vi "image recorder main panel.vi"() -> ()   [LabVIEW 2021]
uses:
  <vilib>/Utility/error.llb/DialogType.ctl
  Image-Stack-Compressor/StackWriterWrapper/LV code/StackWriterWrapper.lvlib
  <vilib>/ptbypt/NI_PtbyPt.lvlib
panel:
  in  "allow long names":bool
  in  "use short dir":bool=TRUE
  out "characters in file name":i32
  in  "Experimenter Name":string
  in  "load control values from file":bool
  in  "save control values to file":bool
  in  "Edit":bool[](array[boolean])
  in  "Add Stimulus":bool
  in  "Delete":bool[](array[boolean])
  out "stimulii":string[](array[string])
  in  "Training/Habituation Pre Exposure":T1
  in  "Stimulus Array":T2(array[cluster])
  in  "Genotype":T3={"GAL4 Line / Line A / Genotype"="CS", "UAS-Effector Line / Line B"=""}
  in  "Project":string
  out "frame add time":u32
  out "last loop time":u32
  in  "left of screen":string="air inlet"
  in  "bottom of screen":string="CS"
  in  "top of screen":string="back of box (y = 0)"
  in  "central region (frac)":dbl caption="central region for placement\nsize (fraction of full screen)"
  out "loop time":u32
  in  "max Background Compression Threads":i32=4
  in  "maxBytesToWrite":u64=1950000000 format="%.2p"
  in  "limit file size?":bool
  out "notes last updated":timestamp format="%<%I:%M %p\n%d/%m/%y>T"
  in  "notes":string
  out "avg frame rate (fps)":dbl
  out "total loop\nwith delay":u32
  out "delay time":dbl
  in  "auto-set":bool
  out "numToWrite":i32(slide) scale=0.0..10.0
  out "numToCompress":i32(slide)=1 scale=0.0..10.0
  out "loop too fast":bool
  in  "min loop time (ms)":u32
  out "timing report":string="-\n  name: adding frame to stack\n  ncalls: 72\n  totaltime: 0.298202\n  maxtime: 0.00436328\n  mintime: 0.00225001\n  avg time: 0.00414169\n  numblowntics: 0\n-\n  name: cloning image\n  ncalls: 72\n  totaltime: 0.24642\n  maxtime: 0.00378184\n  mintime: 0.0017782\n  avg time: 0.0034225\n  numblowntics: 0\n-\n  name: compressing a frame\n  ncalls: 72\n  totaltime: 1.94123\n  maxtime: 0.0403699\n  mintime: 0.0239481\n  avg time: 0.0269615\n  numblowntics: 0\n-\n  name: creating save description\n  ncalls: 1\n  totaltime: 6.19014e-005\n  maxtime: 6.19014e-005\n  mintime: 6.19014e-005\n  avg time: 6.19014e-005\n  numblowntics: 0\n-\n  name: deleting written stack from memory\n  ncalls: 1\n  totaltime: 0.00222322\n  maxtime: 0.00222322\n  mintime: 0.00222322\n  avg time: 0.00222322\n  numblowntics: 0\n-\n  name: writing a stack to disk\n  ncalls: 1\n  totaltime: 0.0259505\n  maxtime: 0.0259505\n  mintime: 0.0259505\n  avg time: 0.0259505\n  numblowntics: 0\ncxcore: 1.0.0, cv: 1.0.0\n\n"
  out "stack destination":string="C:\\data\\test\\t10\\n#n#n#n\\CS(CS)\\2011\\09\\14\\1334\\CS@CS@t10@n#n#n#n@30.mmf"
  out "stackwriter pointer":u32=314603384
  out "loop iteration":i32=23494
  out "error out":errorcluster
  out "maximum loop time":u32
  out "average loop time":dbl format="%.2p"
  in  "max stack size":dbl=1.99
  out "GB written":dbl format="%.2f"
  out "max file size in GB":u64=8589934591
  out "MB written":i32
  out "average time to compress a frame":dbl format="%#_3p"
  out "average time to add a frame to stack":dbl format="%#_3p"
  out "average time to write a stack":dbl format="%#_3p"
  out "elapsed time(s)":dbl
  in  "anticipated frame rate":dbl=30.0
  in  "lgDimMinSize":i32=5
  in  "keyFrameInterval":i32=90
  in  "smallDimMinSize":i32=3
  in  "thresholdAboveBackground":i32=7
  out "buffer number":u32
  in  "base directory":path=path "C:/data/test"
  out "filename":string="CS@CS@t10@n#n#n#n@30"
  out "data directory":path=path "C:/data/test/t10/n#n#n#n/CS(CS)/2011/09/14/1334"
  in  "setup camera?":bool
  in  "STOP PROGRAM":bool
  in  "STOP ACQUISITION":bool
  in  "MAKE DIRECTORIES":bool
  in  "START ACQUISITION":bool
  in  "use ROI":bool
  in  "region of interest":cluster{"x0":u32, "y0":u32, "w":u32, "h":u32}={"x0"=0, "y0"=0, "w"=5000, "h"=5000}
  in  "Acquisiton Time (s)":dbl=660.0
  in  "update image every __ ms":u16=500
  out "Camera Image":T4(plugin-control)
  in  "set all control values as default":bool
  out "GAL4 Line":string="CS"
  # "to reset to actual defaults, delete file\nimage recorder main panel ctl values.dflt"
  # "MMF compression settings"
  # "debugging stuff"
  # "X"
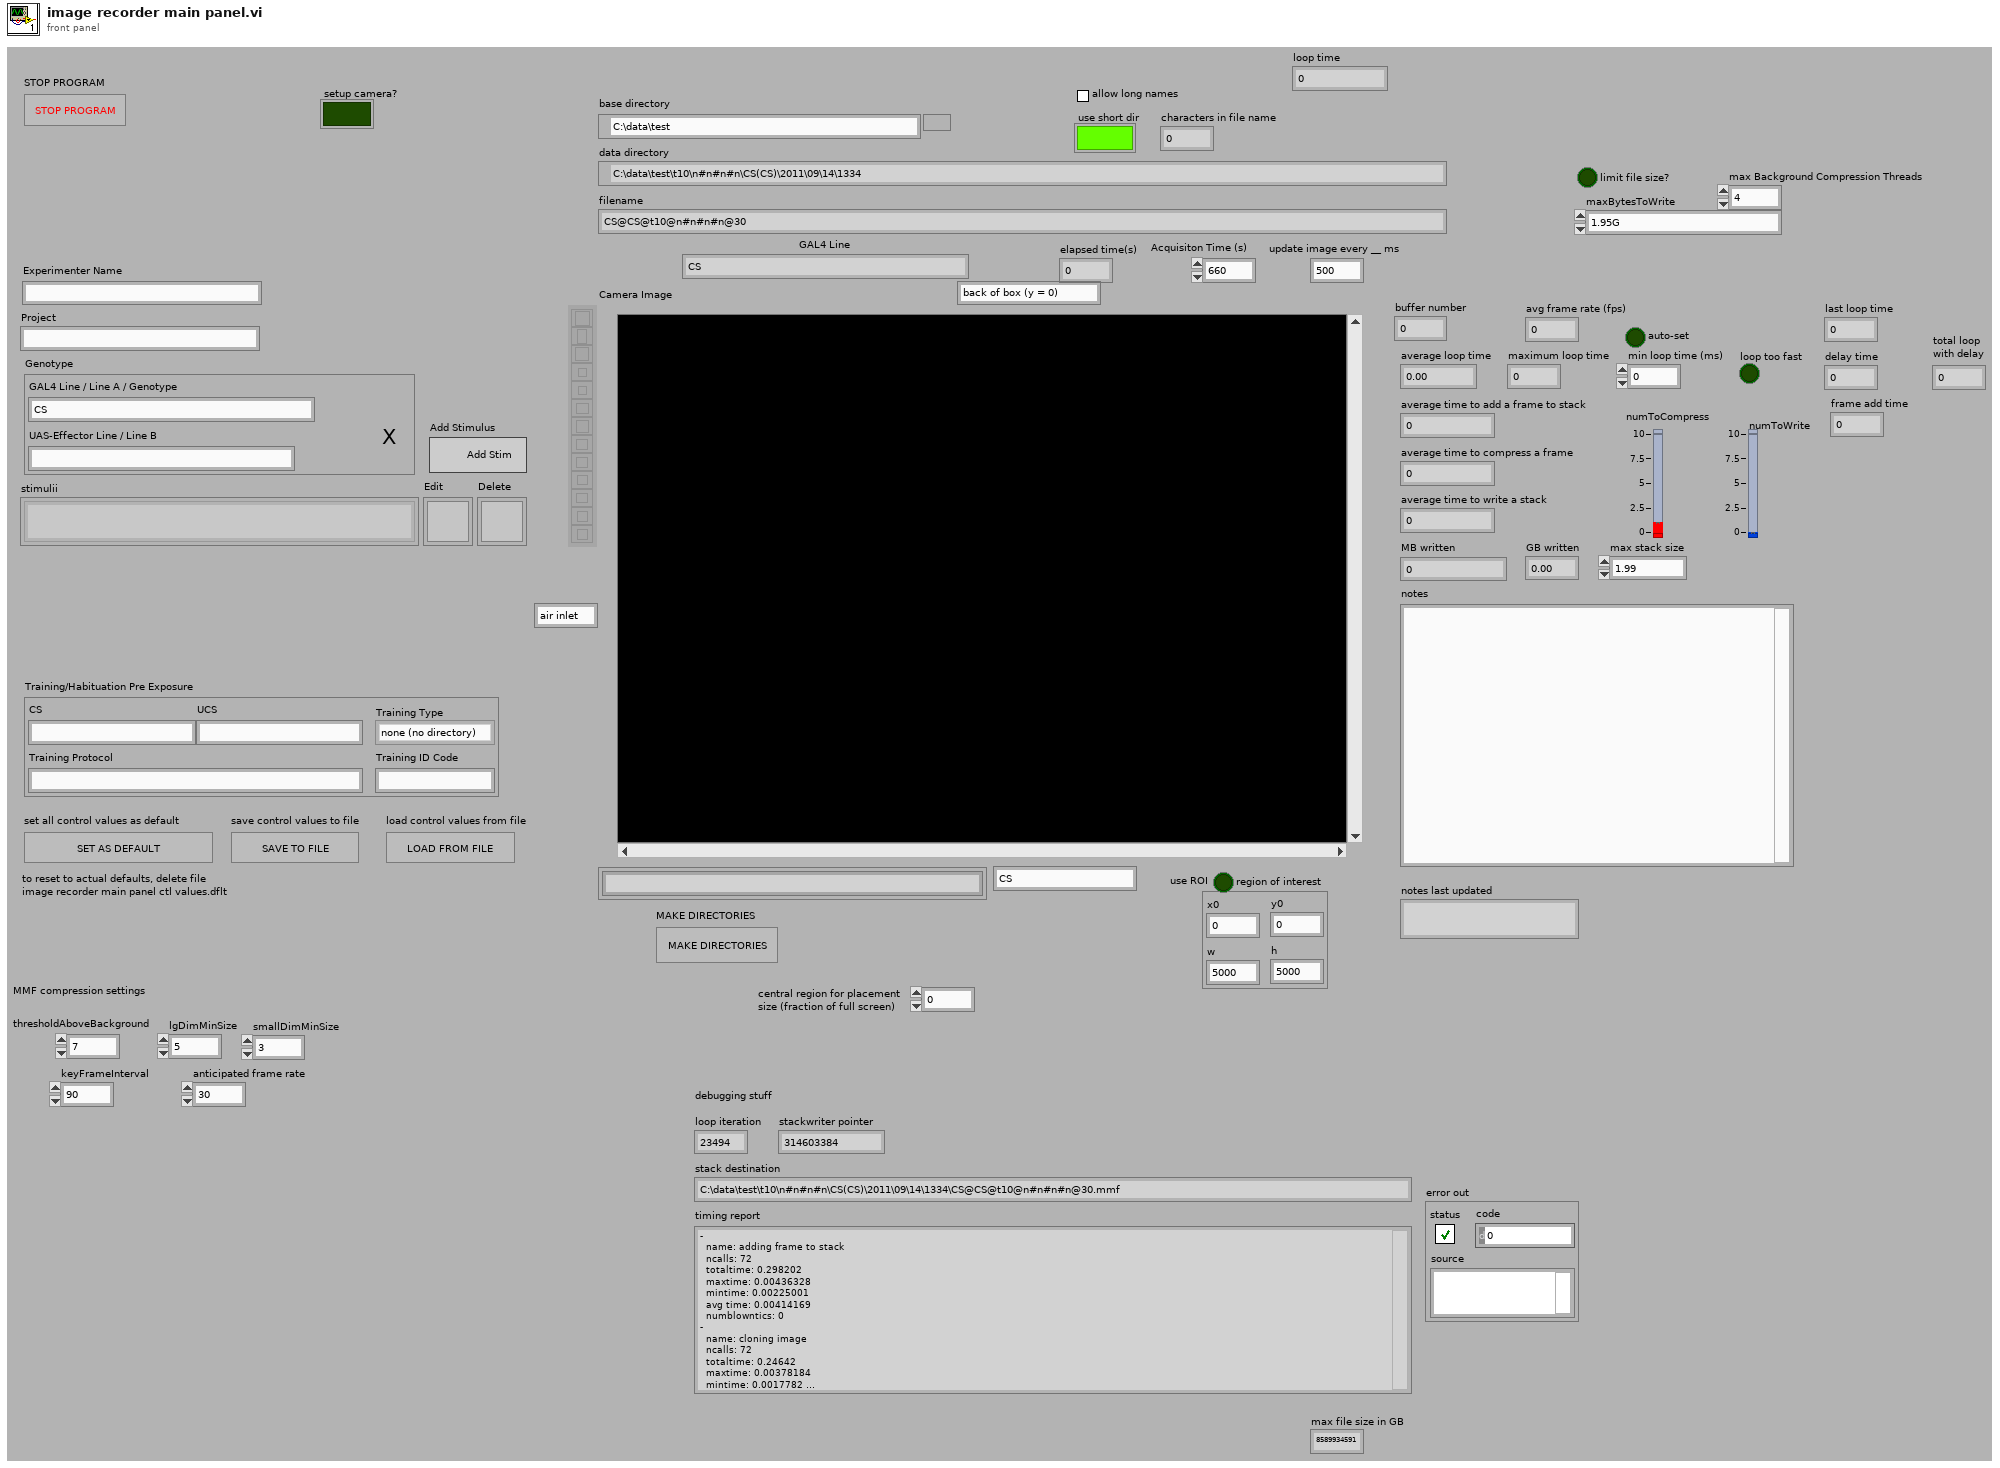
[diagram p1: front panel]
types:
  T1 = cluster{"CS":string, "UCS":string, "Training Protocol":string, "Training ID Code":string, "Training Type":enum16{"none (no directory)", "habituated", "mock habituated", "untrained", "trained"}}
  T2 = cluster{"Stimulus Structure":enum16{"Noise", "Temporal", "Spatial", "Constant", "Other"}, "Stimulant":enum16{"Red Light", "Blue Light", "Green Light", "Odor", "Temperature", "Taste", "Other"}, "Stimulant - additional detail":string, "Noise Parameters":cluster{"Min Val":dbl, "Noise Type":enum16{"Brownian", "Gaussian", "M-Sequence", "Integral of M-Sequence", "Bernoulli", "Uniform", "Other"}, "Max Val":dbl, "Sigma \n(For Gaussian/Brownian)":dbl, "Update Rate (Hz)":dbl, "Full Scale Intensity \n(detector Watts)":dbl, "additional string to append":string, "Other Noise Type":string}, "Temporal Parameters":cluster{"maximum":dbl, "mimimum":dbl, "period (s)":dbl, "Temporal Pattern":enum16{"Triangle", "Sine", "Square", "Other"}, "unit":string, "additional string to append":string, "other pattern":string}, "Spatial Parameters":cluster{"maximum":dbl, "mimimum":dbl, "distance":dbl, "Spatial Pattern":enum16{"XLinear", "YLinear", "Droplet", "Radial", "Other"}, "unit":string, "period_unit":string, "additional string to append":string, "other pattern":string}, "Constant Parameters":cluster{"Value":dbl, "unit":string, "additional string to append":string}, "Other Parameters":cluster{"Long Description of Stimulus And Parameters":string, "Short Description for File Name":string}}[]
  T3 = cluster{"GAL4 Line / Line A / Genotype":string, "UAS-Effector Line / Line B":string}
  T4 = typedef "IMAQ Image.ctl" = refnum<image>
  T5 = typedef "DialogType.ctl" = u16
  T6 = typedef "IMAQdx.ctl" = refnum<k21>
  T7 = cluster{"Aquisition Type":enum16{"IMAQ", "IMAQdx", "AVI", "MMF", "STACK"}, "Interface Name":string, "use roi":bool, "ROI":cluster{"left":u16, "top":u16, "width":u16, "height":u16}, "camera name":T6, "AVI Path":path, "mmf path":path, "stub":string, "Field Width (0 disables 0 padding)":u8, "extension":string, "inter-frame interval (ms)":dbl}
  T8 = typedef "AviRefnum.ctl" = refnum<k1>
  T9 = cluster{"Aquisition Type":enum16{"IMAQ", "IMAQdx", "AVI", "MMF", "STACK"}, "IMAQ Session Out":refnum<k11>, "imaqdx session":T6, "AVI parameters":cluster{"Avi Refnum ":T8, "inter-frame interval (ms)":dbl}, "mmf parameters":cluster{"mmf pointer":u32, "inter-frame interval (ms)":dbl}, "stack read info":cluster{"file stub":string, "format string":string, "extension":string, "inter-frame interval (ms)":dbl}, "camera image":T4, "camera image is 8 bit":bool, "8 bit camera image":T4}
  T10 = enum16{"Reset Table", "Get Values", "Add Value", "Get Table", "Get Spreadsheet", "set stack writer"}
  T11 = enum16{"open", "replace", "create", "open or create", "replace or create", "replace or create with confirmation"}
  T12 = cluster{"Stimulus Structure":enum16{"Noise", "Temporal", "Spatial", "Constant", "Other"}, "Stimulant":enum16{"Red Light", "Blue Light", "Green Light", "Odor", "Temperature", "Taste", "Other"}, "Stimulant - additional detail":string, "Noise Parameters":cluster{"Min Val":dbl, "Noise Type":enum16{"Brownian", "Gaussian", "M-Sequence", "Integral of M-Sequence", "Bernoulli", "Uniform", "Other"}, "Max Val":dbl, "Sigma \n(For Gaussian/Brownian)":dbl, "Update Rate (Hz)":dbl, "Full Scale Intensity \n(detector Watts)":dbl, "additional string to append":string, "Other Noise Type":string}, "Temporal Parameters":cluster{"maximum":dbl, "mimimum":dbl, "period (s)":dbl, "Temporal Pattern":enum16{"Triangle", "Sine", "Square", "Other"}, "unit":string, "additional string to append":string, "other pattern":string}, "Spatial Parameters":cluster{"maximum":dbl, "mimimum":dbl, "distance":dbl, "Spatial Pattern":enum16{"XLinear", "YLinear", "Droplet", "Radial", "Other"}, "unit":string, "period_unit":string, "additional string to append":string, "other pattern":string}, "Constant Parameters":cluster{"Value":dbl, "unit":string, "additional string to append":string}, "Other Parameters":cluster{"Long Description of Stimulus And Parameters":string, "Short Description for File Name":string}}
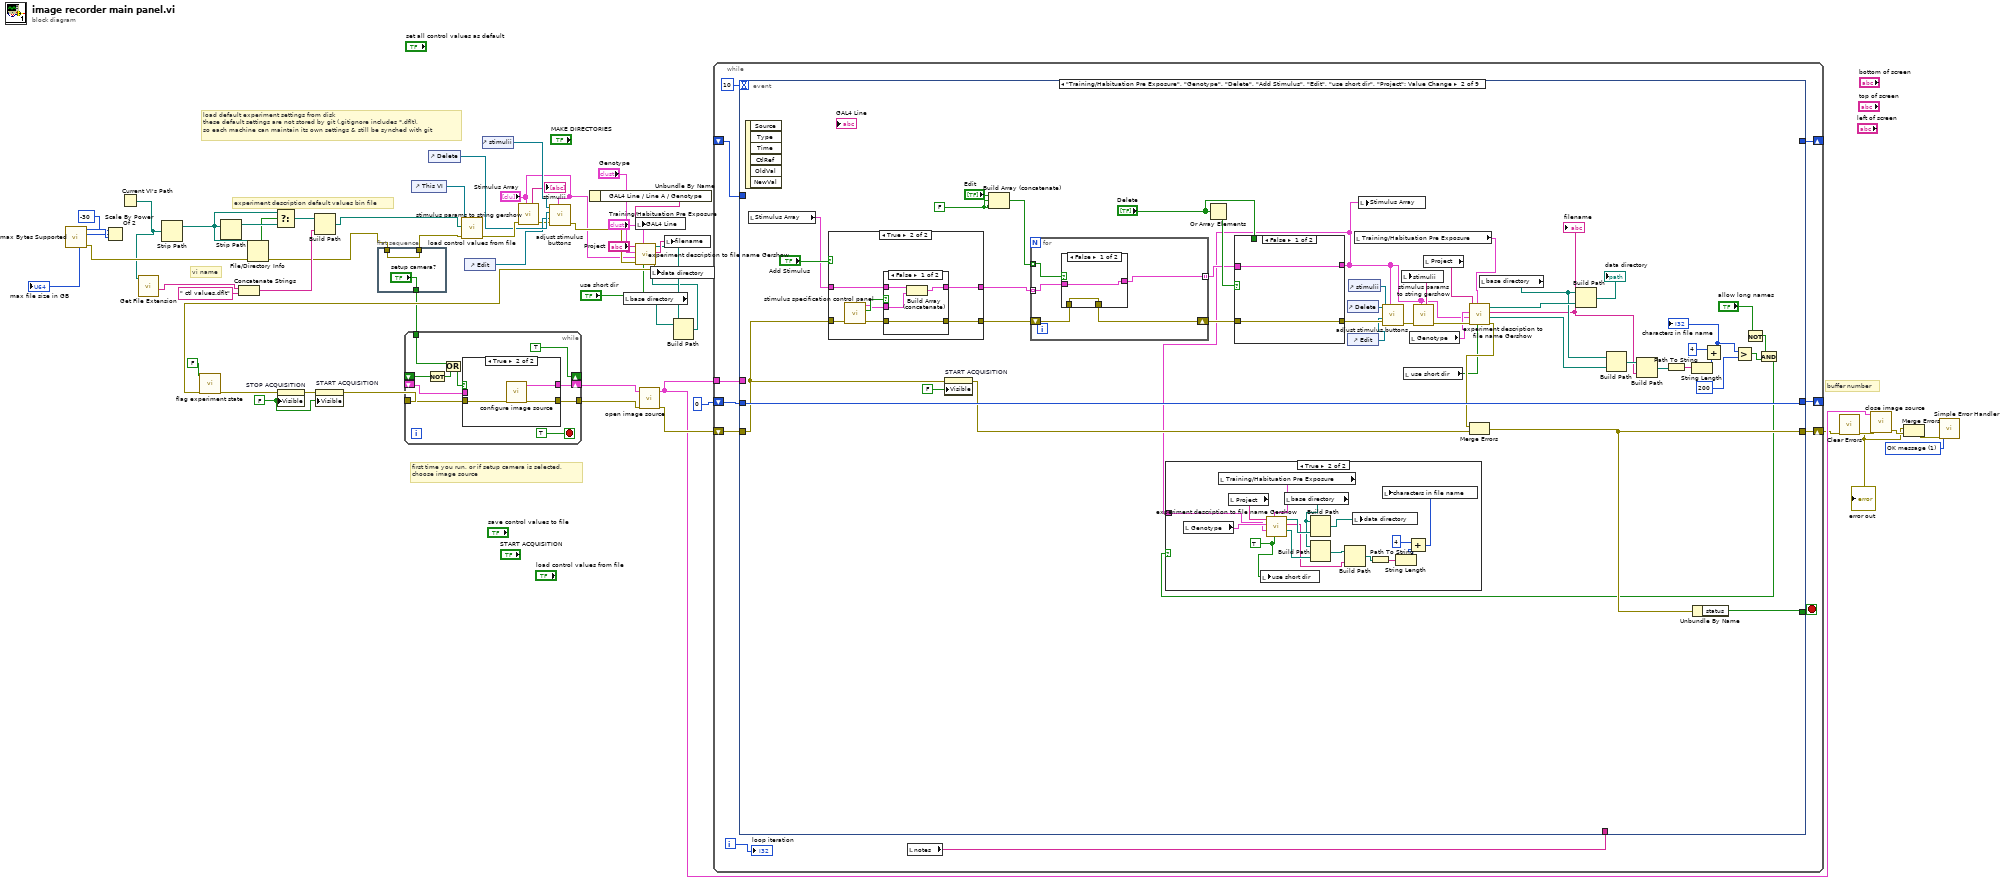
[diagram p0: block diagram]
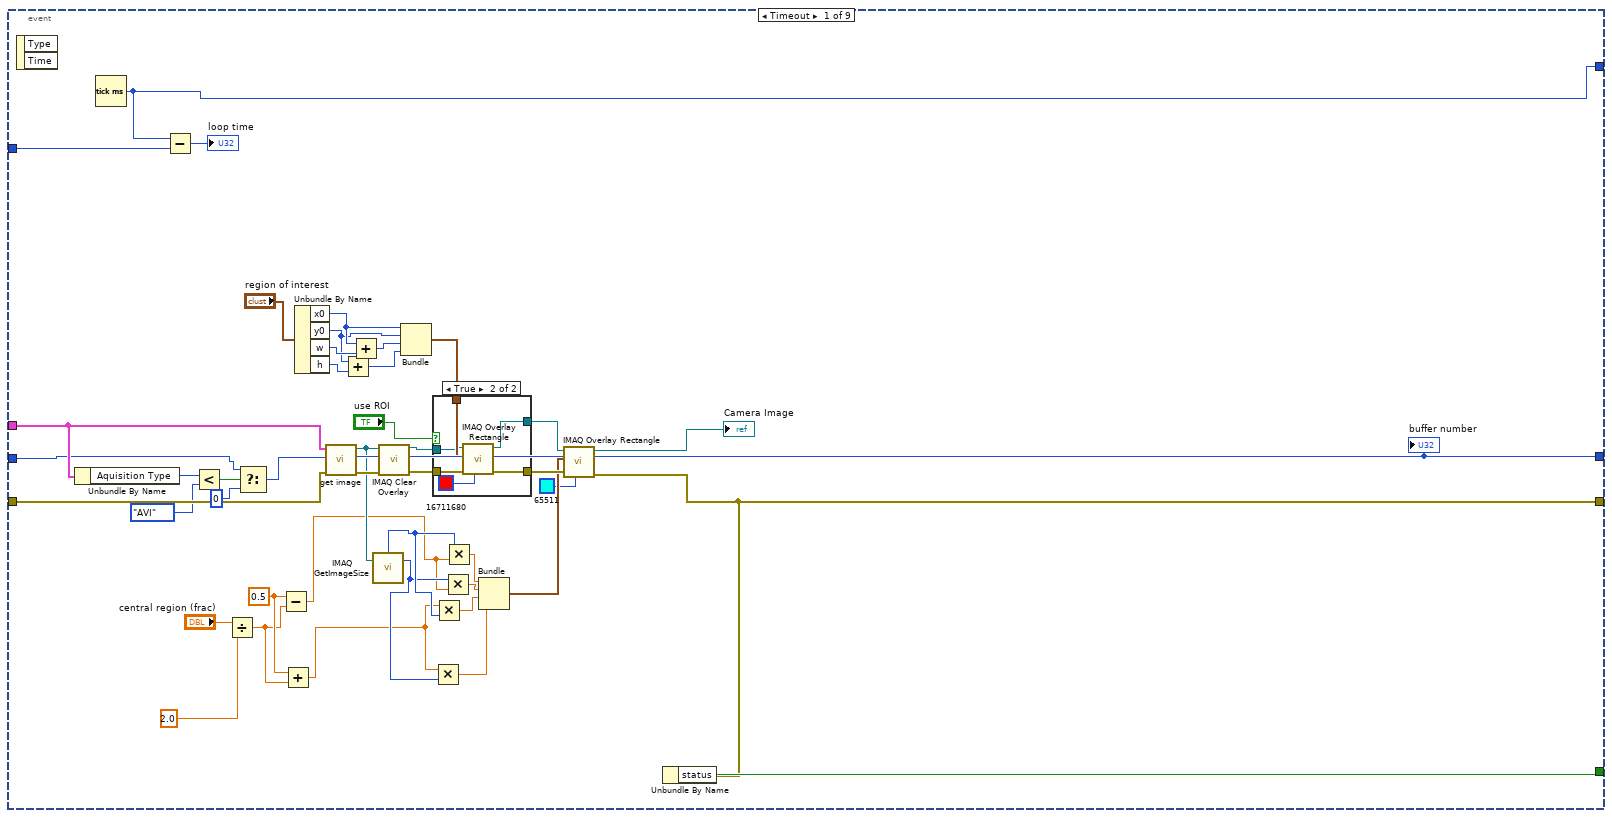
[diagram p3: hidden frame]
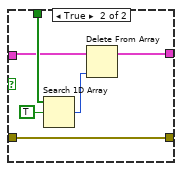
[diagram p6: hidden frame]
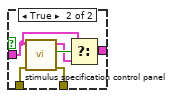
[diagram p7: hidden frame]
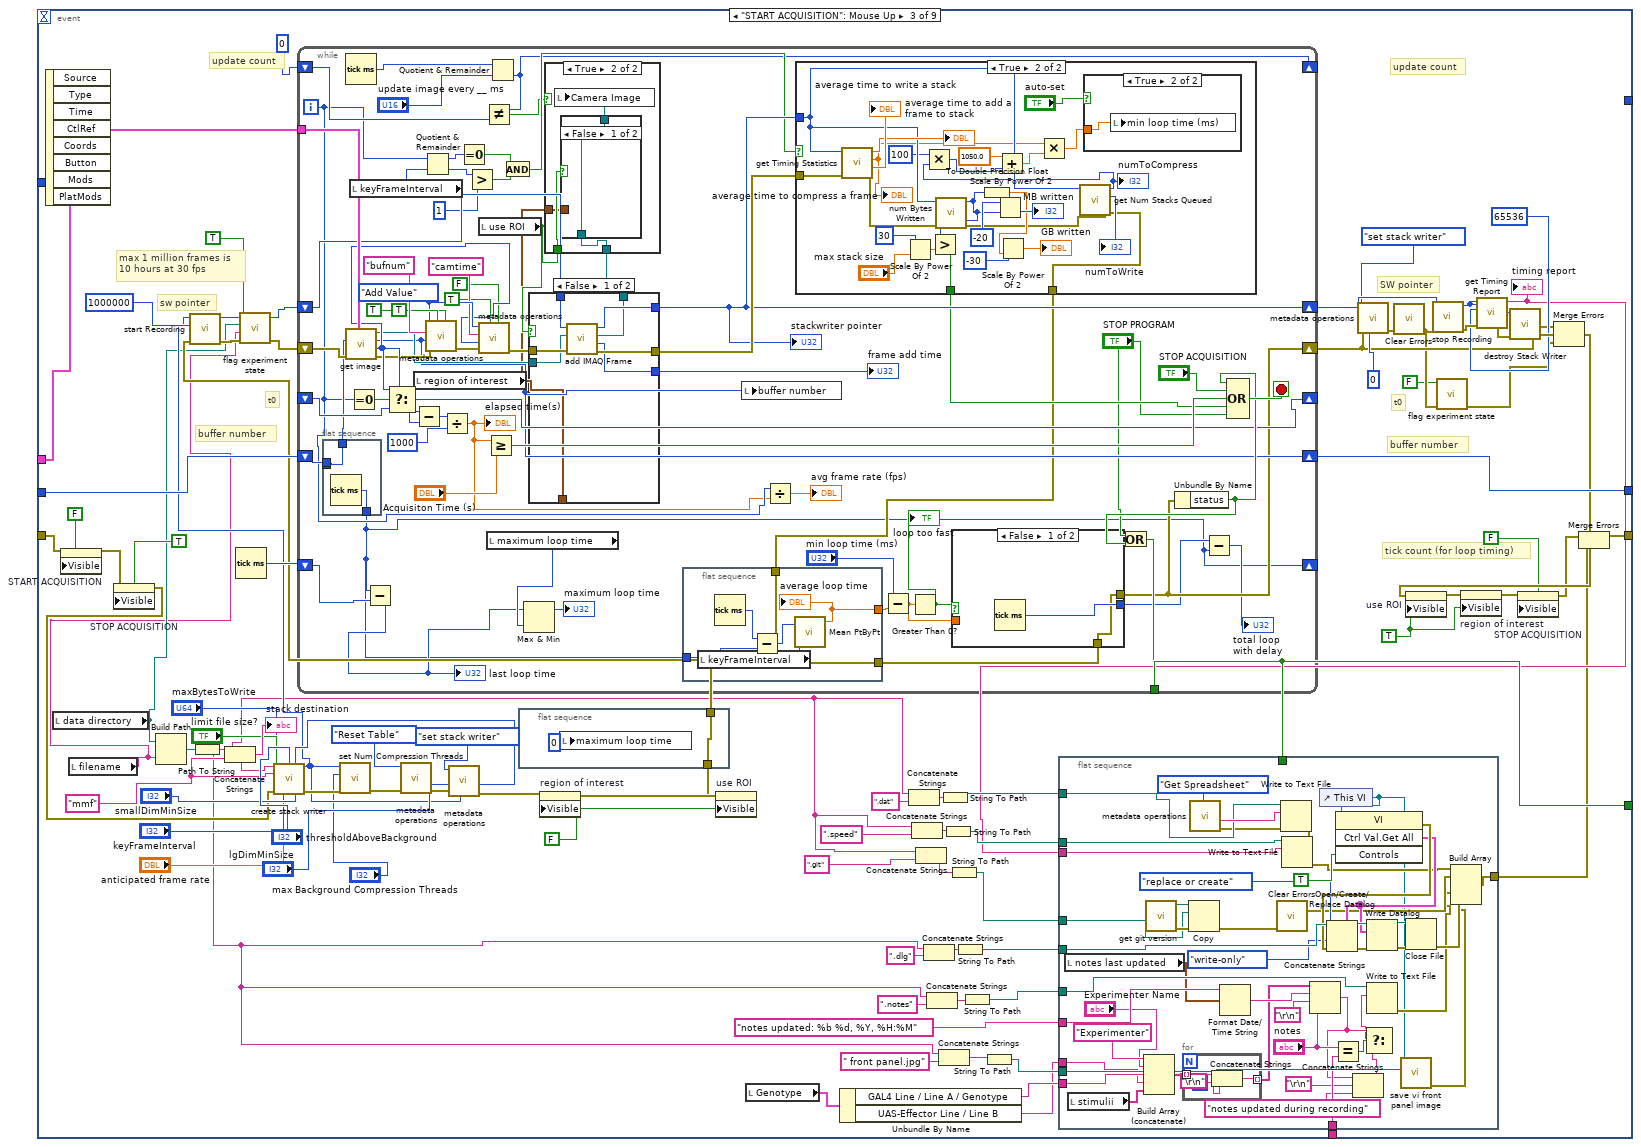
[diagram p10: hidden frame]
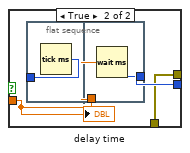
[diagram p11: hidden frame]
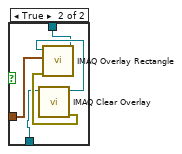
[diagram p13: hidden frame]
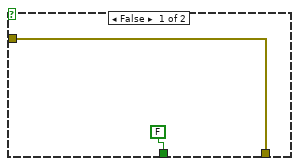
[diagram p14: hidden frame]
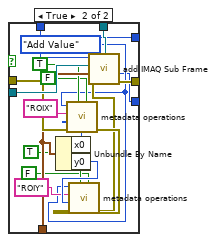
[diagram p16: hidden frame]
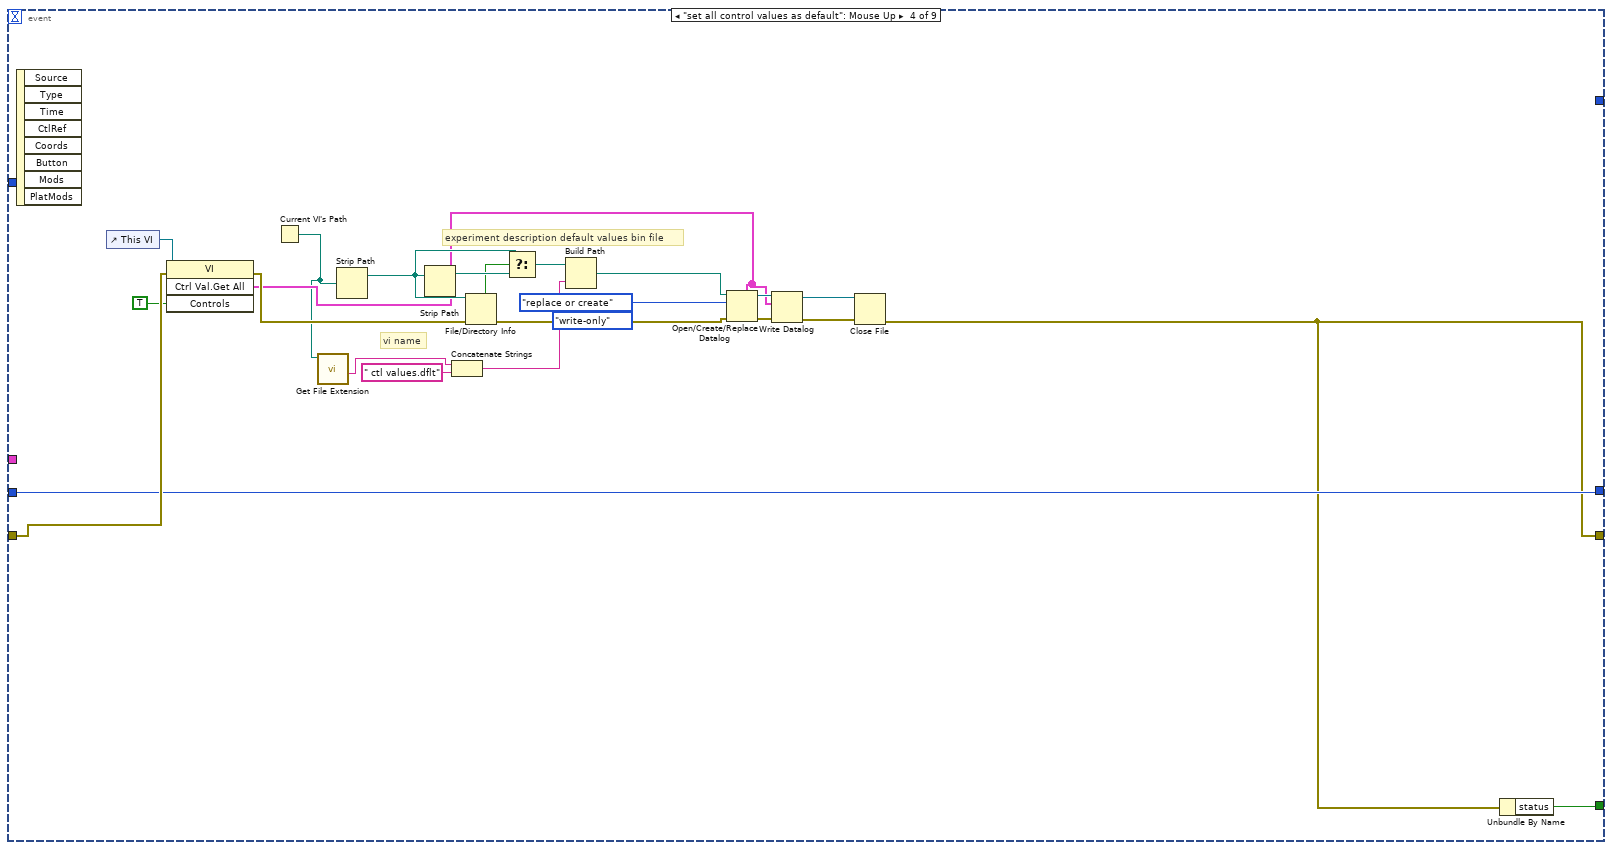
[diagram p17: hidden frame]
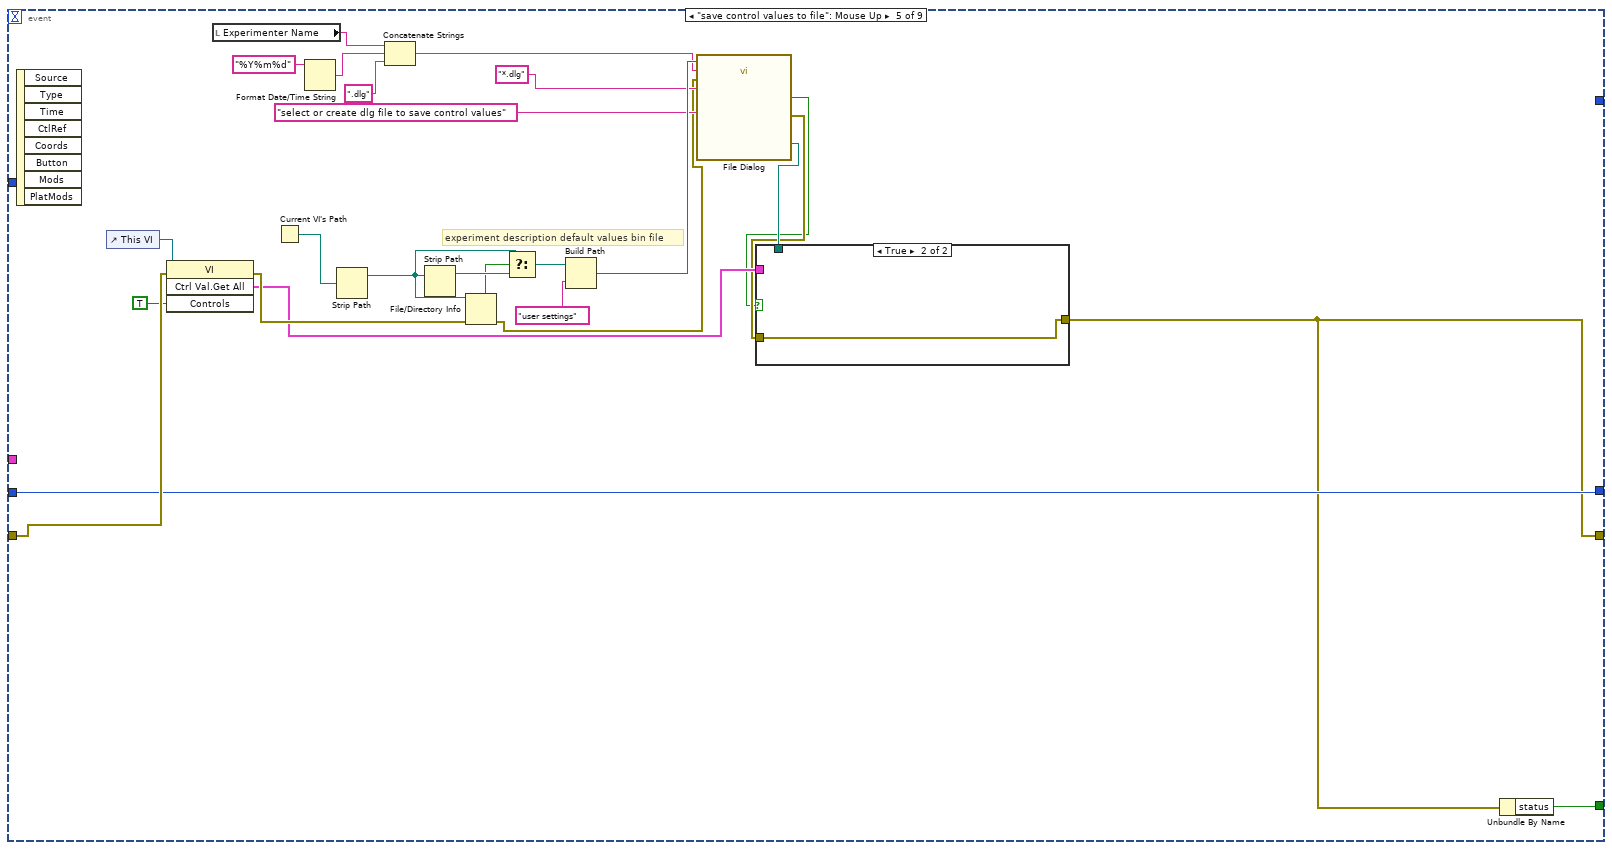
[diagram p18: hidden frame]
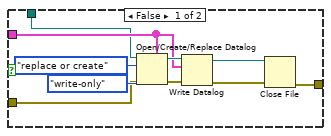
[diagram p19: hidden frame]
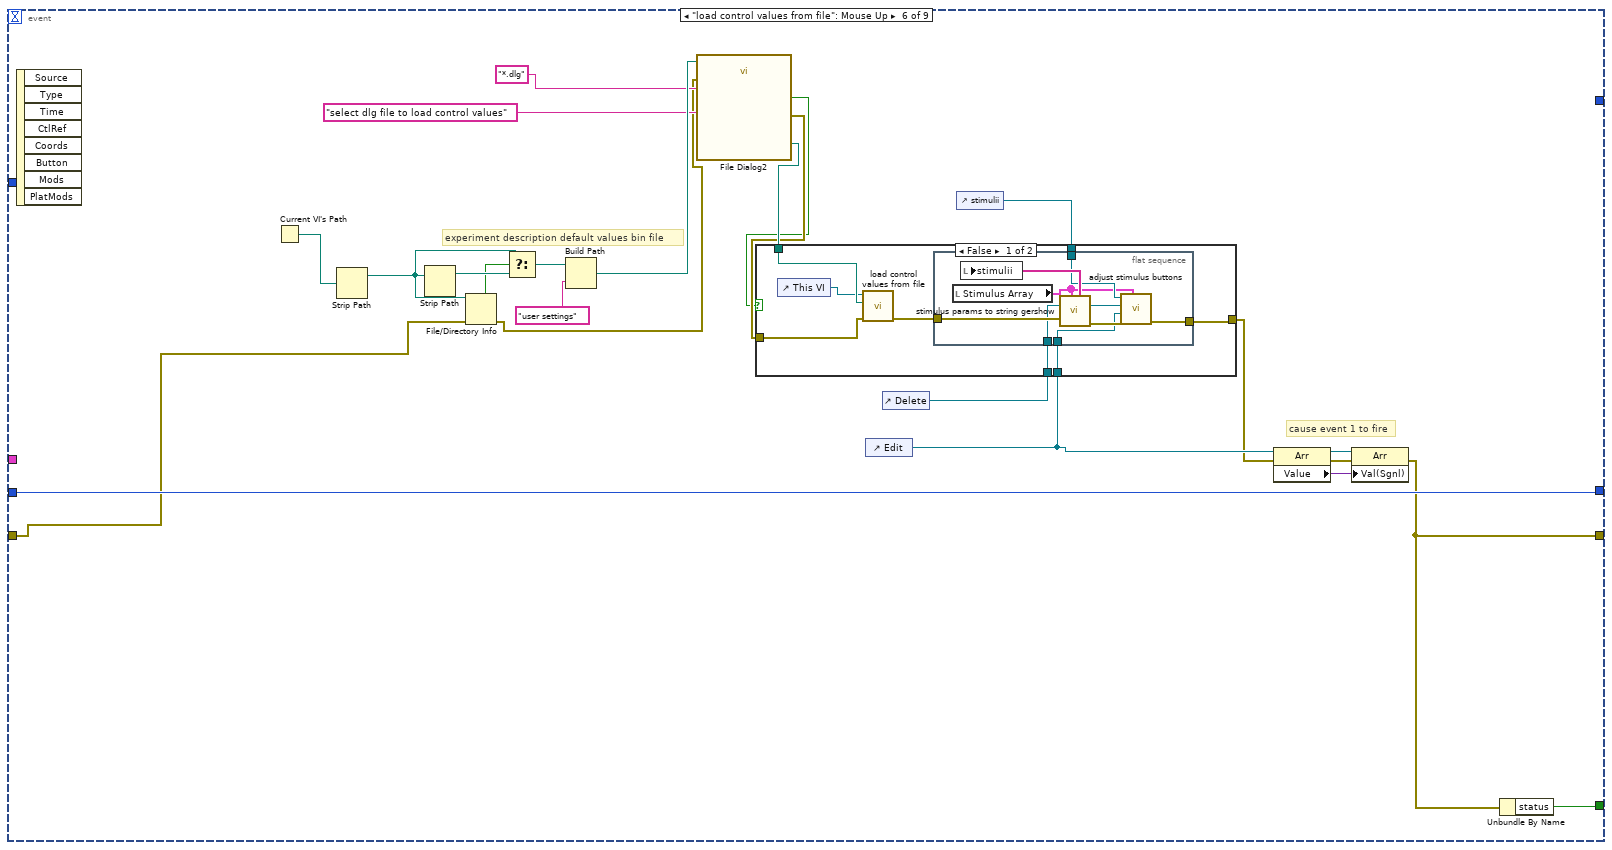
[diagram p20: hidden frame]
diagram:
  w26 = T5 1 items=["no dialog", "OK message", "continue or stop message", "OK message + warnings", "continue/stop + warnings"] ("type of dialog (OK msg:1)")
  w38 = FALSE ("Visible")
  # "buffer number"
  # "first time you run, or if setup camera is selected, \nchoose image source"
  # "load default experiment settings from disk\nthese default settings are not stored by git (.gitignore includes *.dflt), \nso each machine can maintain its own settings & still be synched with git"
  # "experiment description default values bin file"
  # "vi name"
  n1 = call "max Bytes Supported.vi"() -> ("error out"=w35:errorcluster, "function return"=w34:u32)  [unwired: 10 in]
  n2 = Scale By Power Of 2(n=-30, x=w34) -> (x*2^n=→"max file size in GB":u32)
  n3 = Current VI's Path() -> (path=w18:path)
  n4 = call <vilib>:"Get File Extension.vi"("file"=w18) -> ("filename without extension"=w17:string)  [unwired: 6 in, 4 out]
  n5 = Strip Path(path=w18) -> (stripped path=w50:path)  [unwired: 1 out]
  n6 = Strip Path(path=w50) -> (stripped path=w49:path)  [unwired: 1 out]
  n7 = Concatenate Strings(w17, " ctl values.dflt" ("string")) -> (w45:string)
  n8 = File/Directory Info(path=w50, error in=w35) -> (directory=w48:bool, error out=w3:errorcluster)  [unwired: 5 out]
  n9 = Select(t=w50, s=w48, f=w49) -> (s? t:f=w46:path)
  n10 = Build Path(base path=w46, name or relative path=w45) -> (appended path=w22:path)
  n11 = flat-sequence {
    tunnel: w3 -> [w52]
    tunnel: [w52] -> w2
    tunnel: ["setup camera?"] -> w1
    frame #0 {
    }
  }
  n12 = control-ref of="This VI"() -> (w19:refnum<vi>)
  n13 = control-ref of="Delete"() -> (w11:refnum<vi>)
  n14 = call "load control values from file.vi"("error in (no error)"=w2, "datalog path (use dialog)"=w22, "VI ref"=w19) -> ("error out"=w21:errorcluster)  [unwired: 8 in]
  n15 = control-ref of="Edit"() -> (w10:refnum<vi>)
  n16 = control-ref of="stimulii"() -> (w12:refnum<vi>)
  n17 = call "stimulus params to string gershow.vi"("Stimulus cluster array"="Stimulus Array", "error in"=w21) -> ("error out"=w6:errorcluster, "long string array"=→"stimulii":string[])  [unwired: 5 in, 3 out]
  n18 = call "adjust stimulus buttons.vi"("Stimulus Array"="Stimulus Array", "error in (no error)"=w6, "Edit handle"=w10, "Delete handle"=w11, "stimulii handle"=w12) -> ("error out"=w9:errorcluster)  [unwired: 6 in]
  n19 = Unbundle By Name("Genotype") -> ("GAL4 Line / Line A / Genotype"=w44:string)
  n20 = local read "base directory"() -> (w25:path)
  n21 = local write "GAL4 Line"(w44) -> ()
  n22 = call "experiment description to file name Gershow.vi"("use short dir"="use short dir", "Training/Habituation Pre Exposure"="Training/Habituation Pre Exposure", "error in"=w9, "Stimulus Array"="Stimulus Array", "Genotype"="Genotype", "Project"="Project") -> ("error out"=w8:errorcluster, "filename"=w36:string, "data directory"=w24:path)  [unwired: 2 in, 1 out]
  n23 = call "flag experiment state.vi"("error in (no error)"=w8, "experiment started"=FALSE) -> ("error out"=w16:errorcluster)  [unwired: 9 in]
  n24 = property on="STOP ACQUISITION" class="Bool"(error in=w16, "Visible"=w38) -> (error out=w39:errorcluster)  [unwired: 1 in, 1 out]
  n25 = property on="START ACQUISITION" class="Bool (strict)"(error in=w39, "Visible"=w38) -> (error out=w37:errorcluster)  [unwired: 1 in, 1 out]
  n26 = while {
    shift-right: [TRUE] -> _
    shift-left: _ -> [w59]
    tunnel: w37 -> [w57]
    tunnel: [w56] -> w42
    shift-right: [w55] -> w43
    shift-left: _ -> [w54]
    tunnel: w1 -> [w53]
    stop <- TRUE stop-if-true
    n27 = Not(x=w59) -> (.not. x?=w58:bool)
    n28 = Or(x=w53, y=w58) -> (x .or. y?=w61:bool)
    n29 = case shown="True" w61 {
      tunnel: w57 -> [w63 w67]
      tunnel: [w63 w66] -> w56
      tunnel: [w64 w65] -> w55
      tunnel: w54 -> [w64 _]
      frame False {
      }
      frame True {
        n30 = call "configure image source.vi"("error in (no error)"=w67) -> ("error out"=w66:errorcluster, "image source parameters"=w65:T7)  [unwired: 9 in]
      }
    }
  }
  n31 = call "open image source.vi"("error in (no error)"=w42, "image source parameters"=w43) -> ("error out"=w41:errorcluster, "image source data"=w31:T9)  [unwired: 8 in]
  n32 = local write "filename"(w36) -> ()
  n33 = Build Path(base path=w25, name or relative path=w24) -> (appended path=w23:path)
  n34 = local write "data directory"(w23) -> ()
  n35 = while {
    shift-right: [w74] -> w28
    shift-left: w41 -> [w77]
    tunnel: w31 -> [w76]
    shift-right: [w73] -> _
    shift-left: 0 -> [w75]
    shift-right: [w70] -> _
    shift-left: _ -> [w69]
    i -> [w72]
    stop <- w78 stop-if-true
    n36 = local read "notes"() -> (w68:string)
    n37 = event shown="[1] \"Training/Habituation Pre Exposure\", \"Genotype\", \"Delete\", \"Add Stimulus\", \"Edit\", \"use short dir\", \"Project\": Value Change" {
      selector: _ -> [_ _ _ _ _ _ _ _ _]
      dyn-events: _ -> [_ _ _ _ _ _ _ _ _]
      timeout: 10 -> [_ _ _ _ _ _ _ _ _]
      tunnel: [w113 w175 w277 w518 w553 w594 TRUE ("status") w630 FALSE ("status")] -> w78
      tunnel: w77 -> [w122 w169 w301 w538 w564 w585 w618 w623 w655]
      tunnel: w76 -> [w121 _ w305 _ _ _ _ _ _]
      tunnel: w75 -> [w117 w176 w307 w520 w555 w595 w620 w631 w654]
      tunnel: [w96 w151 w260 w519 w554 w578 w618 w629 w655] -> w74
      tunnel: [w114 w176 w306 w520 w555 w595 w620 w631 w654] -> w73
      tunnel: [w99 _ _ _ _ _ _ _ _] -> w70
      tunnel: w69 -> [w100 _ _ _ _ _ _ _ _]
      tunnel: w68 -> [_ _ w229 _ _ _ _ _ _]
      event Timeout {
        w84 = 0.5 ("x")
        n38 = event-data() -> ()  [unwired: 1 in, 2 out]
        n39 = Unbundle By Name(w121) -> ("Aquisition Type"=w120:enum16{"IMAQ", "IMAQdx", "AVI", "MMF", "STACK"})
        n40 = Tick Count (ms)() -> (millisecond timer value=w99:u32)
        n41 = Subtract(x=w99, y=w100) -> (x-y=→"loop time":u32)
        n42 = Less?(x=w120, y=enum16{"IMAQ", "IMAQdx", "AVI", "MMF", "STACK"}."AVI") -> (x < y?=w118:bool)
        n43 = Divide(x="central region (frac)", y=2.0) -> (x/y=w81:dbl)
        n44 = Select(t=w117, s=w118, f=0) -> (s? t:f=w115:u32)
        n45 = Subtract(x=w84, y=w81) -> (x-y=w80:dbl)
        n46 = Add(x=w84, y=w81) -> (x+y=w79:dbl)
        n47 = Unbundle By Name("region of interest") -> ("x0"=w107:u32, "y0"=w106:u32, "w"=w109:u32, "h"=w108:u32)
        n48 = call "get image.vi"("error in (no error)"=w122, "previous buffer number"=w115, "image source data"=w121) -> ("error out"=w112:errorcluster, "buffer number"=w114:u32, "captured image"=w93:T4)  [unwired: 5 in, 1 out]
        "buffer number" <- w114
        n49 = Add(x=w106, y=w108) -> (x+y=w104:u32)
        n50 = Add(x=w107, y=w109) -> (x+y=w105:u32)
        n51 = call "IMAQ GetImageSize"("Image"=w93) -> ("Y Resolution"=w89:i32, "X Resolution"=w90:i32)  [unwired: 3 in, 1 out]
        n52 = call "IMAQ Clear Overlay"("error in (no error)"=w112, "Image"=w93) -> ("error out"=w101:errorcluster, "Image Out"=w102:T4)  [unwired: 8 in]
        n53 = Bundle("x0"=w107, "y0"=w106, w105, w104) -> (w103:cluster{"x0":u32, "y0":u32, u32, u32})  [unwired: 1 in]
        n54 = case shown="True" "use ROI" {
          tunnel: w103 -> [_ w130]
          tunnel: w102 -> [w124 w129]
          tunnel: w101 -> [w123 w128]
          tunnel: [w124 w126] -> w94
          tunnel: [w123 w125] -> w97
          frame False {
          }
          frame True {
            n55 = call "IMAQ Overlay Rectangle"("Color"=u32 16711680, "error in (no error)"=w128, "Rectangle"=w130, "Image"=w129) -> ("error out"=w125:errorcluster, "Image Out"=w126:T4)  [unwired: 6 in]
          }
        }
        n56 = Multiply(x=w79, y=w89) -> (x*y=w87:dbl)
        n57 = Multiply(x=w79, y=w90) -> (x*y=w88:dbl)
        n58 = Multiply(x=w89, y=w80) -> (x*y=w91:dbl)
        n59 = Multiply(x=w90, y=w80) -> (x*y=w92:dbl)
        n60 = Bundle(w92, w91, w88, w87) -> (w86:cluster{dbl, dbl, dbl, dbl})  [unwired: 1 in]
        n61 = call "IMAQ Overlay Rectangle"("Color"=u32 65511, "error in (no error)"=w97, "Rectangle"=w86, "Image"=w94) -> ("error out"=w96:errorcluster, "Image Out"=→"Camera Image":T4)  [unwired: 6 in]
        n62 = Unbundle By Name(w96) -> ("status"=w113:bool)
      }
      event "Training/Habituation Pre Exposure", "Genotype", "Delete", "Add Stimulus", "Edit", "use short dir", "Project": Value Change {
        w147 = FALSE ("logical OR")
        n63 = event-data() -> ()  [unwired: 1 in, 6 out]
        n64 = local read "Stimulus Array"() -> (w168:T2)
        n65 = case shown="True" "Add Stimulus" {
          tunnel: w169 -> [w214 w222]
          tunnel: w168 -> [w215 w220]
          tunnel: [w215 w219] -> w149
          tunnel: [w214 w216] -> w166
          frame False {
          }
          frame True {
            n66 = call "stimulus specification control panel.vi"("error in"=w222) -> ("error out"=w217:errorcluster, "canceled?"=w221:bool, "Stimulus Cluster Out"=w218:T12)  [unwired: 8 in]
            n67 = case shown="False" w221 {
              tunnel: w220 -> [w226 w228]
              tunnel: [w224 w228] -> w219
              tunnel: w218 -> [w225 _]
              tunnel: w217 -> [w223 w227]
              tunnel: [w223 w227] -> w216
              frame False {
                n68 = Build Array (concatenate)(w226, w225) -> (w224:T2)
              }
              frame True {
              }
            }
          }
        }
        n69 = property on="START ACQUISITION" class="Bool (strict)"(error in=w169, "Visible"=FALSE) -> (error out=w173:errorcluster)  [unwired: 1 in, 1 out]
        n70 = Build Array (concatenate)("Edit", w147, w147) -> (w148:bool[])
        n71 = for {
          tunnel: w149 -> [w203] mode=indexing
          tunnel: w148 -> [w204] mode=indexing
          shift-right: [w202] -> w164
          shift-left: w166 -> [w205]
          tunnel: [w201] -> w163 mode=indexing
          n72 = case shown="False" w204 {
            tunnel: w205 -> [w207 w213]
            tunnel: w203 -> [w206 w209]
            tunnel: [w207 w212] -> w202
            tunnel: [w206 w208] -> w201
            frame False {
            }
            frame True {
              n73 = call "stimulus specification control panel.vi"("error in"=w213, "Stimulus Cluster In"=w209) -> ("error out"=w212:errorcluster, "canceled?"=w211:bool, "Stimulus Cluster Out"=w210:T12)  [unwired: 7 in]
              n74 = Select(t=w209, s=w211, f=w210) -> (s? t:f=w208:T12)
            }
          }
        }
        n75 = Or Array Elements(Boolean array="Delete") -> (logical OR=w165:bool)
        n76 = case shown="False" w165 {
          tunnel: w164 -> [w193 w195]
          tunnel: w163 -> [w194 w198]
          tunnel: "Delete" -> [_ w200]
          tunnel: [w194 w196] -> w134
          tunnel: [w193 w195] -> w161
          frame False {
          }
          frame True {
            n77 = Search 1D Array(1D array=w200, element=TRUE) -> (index of element=w197:i32)  [unwired: 1 in]
            n78 = Delete From Array(array=w198, index=w197) -> (array with subset deleted=w196:T2)  [unwired: 1 in, 1 out]
          }
        }
        n79 = control-ref of="Delete"() -> (w159:refnum<vi>)
        n80 = control-ref of="Edit"() -> (w158:refnum<vi>)
        n81 = control-ref of="stimulii"() -> (w160:refnum<vi>)
        n82 = local read "Training/Habituation Pre Exposure"() -> (w152:T1)
        n83 = local write "Stimulus Array"(w134) -> ()
        n84 = call "adjust stimulus buttons.vi"("Stimulus Array"=w134, "error in (no error)"=w161, "Edit handle"=w158, "Delete handle"=w159, "stimulii handle"=w160) -> ("error out"=w157:errorcluster)  [unwired: 6 in]
        n85 = local read "use short dir"() -> (w135:bool)
        n86 = local read "Genotype"() -> (w154:T3)
        n87 = call "stimulus params to string gershow.vi"("Stimulus cluster array"=w134, "error in"=w157) -> ("error out"=w155:errorcluster, "long string array"=w156:string[])  [unwired: 5 in, 3 out]
        n88 = local write "stimulii"(w156) -> ()
        n89 = local read "Project"() -> (w153:string)
        n90 = call "experiment description to file name Gershow.vi"("use short dir"=w135, "Training/Habituation Pre Exposure"=w152, "error in"=w155, "Stimulus Array"=w134, "Genotype"=w154, "Project"=w153) -> ("error out"=w150:errorcluster, "data directory with time"=w146:path, "filename"=w143:string, "data directory"=w172:path)  [unwired: 2 in]
        "filename" <- w143
        n91 = Merge Errors(w150, w173) -> (w151:errorcluster)
        n92 = local read "base directory"() -> (w145:path)
        n93 = Build Path(base path=w145, name or relative path=w172) -> (appended path=→"data directory":path)
        n94 = Build Path(base path=w145, name or relative path=w146) -> (appended path=w144:path)
        n95 = Build Path(base path=w144, name or relative path=w143) -> (appended path=w142:path)
        n96 = Path To String(path=w142) -> (string=w141:string)
        n97 = String Length(string=w141) -> (length=w140:i32)
        n98 = Unbundle By Name(w151) -> ("status"=w175:bool)
        n99 = Add(x=4, y=w140) -> (x+y=w138:i32)
        "characters in file name" <- w138
        n100 = Greater?(x=w138, y=200) -> (0:w136:bool)
        n101 = Not(x="allow long names") -> (.not. x?=w132:bool)
        n102 = And(x=w132, y=w136) -> (x .and. y?=w133:bool)
        n103 = case shown="True" w133 {
          tunnel: w134 -> [_ w188]
          frame False {
          }
          frame True {
            w192 = TRUE ("use short dir")
            n104 = local read "Genotype"() -> (w189:T3)
            n105 = local read "Training/Habituation Pre Exposure"() -> (w190:T1)
            n106 = local read "Project"() -> (w191:string)
            n107 = local write "use short dir"(w192) -> ()
            n108 = call "experiment description to file name Gershow.vi"("use short dir"=w192, "Training/Habituation Pre Exposure"=w190, "Stimulus Array"=w188, "Genotype"=w189, "Project"=w191) -> ("data directory with time"=w184:path, "filename"=w182:string, "data directory"=w186:path)  [unwired: 3 in, 1 out]
            n109 = local read "base directory"() -> (w185:path)
            n110 = Build Path(base path=w185, name or relative path=w186) -> (appended path=w187:path)
            n111 = Build Path(base path=w185, name or relative path=w184) -> (appended path=w183:path)
            n112 = Build Path(base path=w183, name or relative path=w182) -> (appended path=w179:path)
            n113 = local write "data directory"(w187) -> ()
            n114 = Path To String(path=w179) -> (string=w181:string)
            n115 = String Length(string=w181) -> (length=w178:i32)
            n116 = Add(x=4, y=w178) -> (x+y=w177:i32)
            n117 = local write "characters in file name"(w177) -> ()
          }
        }
      }
      event "START ACQUISITION": Mouse Up {
        w283 = TRUE ("Visible")
        w293 = FALSE ("Visible")
        w244 = "mmf" ("string")
        # "tick count (for loop timing)"
        # "max 1 million frames is \n10 hours at 30 fps"
        # "update count"
        # "buffer number"
        # "t0"
        # "update count"
        # "sw pointer"
        # "buffer number"
        # "t0"
        # "SW pointer"
        n118 = event-data() -> ()  [unwired: 1 in, 8 out]
        n119 = local read "data directory"() -> (w238:path)
        n120 = property on="START ACQUISITION" class="Bool (strict)"(error in=w301, "Visible"=FALSE) -> (error out=w303:errorcluster)  [unwired: 1 in, 1 out]
        n121 = local read "filename"() -> (w237:string)
        n122 = property on="STOP ACQUISITION" class="Bool"(error in=w303, "Visible"=TRUE) -> (error out=w300:errorcluster)  [unwired: 1 in, 1 out]
        n123 = Build Path(base path=w238, name or relative path=w237) -> (appended path=w314:path)
        n124 = Path To String(path=w314) -> (string=w236:string)
        n125 = Concatenate Strings(w236, w244) -> (→"stack destination":string)
        n126 = Tick Count (ms)() -> (millisecond timer value=w287:u32)
        n127 = call "create stack writer.vi"("file stub"=w236, "keyFrameInterval"="keyFrameInterval", "thresholdAboveBackground"="thresholdAboveBackground", "lgDimMinSize"="lgDimMinSize", "extension"=w244, "limit file size?"="limit file size?", "maxBytesToWrite"="maxBytesToWrite", "error in (no error)"=w300, "anticipated frame rate"="anticipated frame rate", "smallDimMinSize"="smallDimMinSize") -> ("stack writer pointer"=w240:u32, "error out"=w296:errorcluster)  [unwired: 4 in]
        n128 = call "start Recording.vi"("error in (no error)"=w285, "nframes"=1000000, "sw"=w240) -> ("error out"=w291:errorcluster, "sw out"=w292:u32)  [unwired: 6 in, 1 out]
        n129 = call "flag experiment state.vi"("error in (no error)"=w291, "filename"=w237, "data directory"=w238, "experiment started"=TRUE) -> ("error out"=w249:errorcluster)  [unwired: 7 in]
        n130 = while {
          shift-right: [w413] -> w254
          shift-left: w292 -> [w417]
          shift-right: [w382] -> w251
          shift-left: w249 -> [w434]
          shift-right: [w390] -> w306
          shift-left: w307 -> [w383]
          shift-right: [w391] -> _
          shift-left: _ -> [w431]
          tunnel: w305 -> [w433]
          shift-right: [w396] -> _
          shift-left: u32 0 -> [w415]
          tunnel: [w405] -> w277
          shift-right: [w371] -> _
          shift-left: w287 -> [w394]
          i -> [w377]
          stop <- w409 stop-if-true
          w426 = T10."Add Value" ("Operation")
          n131 = flat-sequence {
            tunnel: [w442] -> w371
            tunnel: [w441] -> w384
            tunnel: [w441] -> _
            tunnel: w383 -> [w441]
            frame #0 {
              n132 = Tick Count (ms)() -> (millisecond timer value=w442:u32)
            }
          }
          n133 = Tick Count (ms)() -> (millisecond timer value=w408:u32)
          n134 = call "get image.vi"("error in (no error)"=w434, "previous buffer number"=w384, "image source data"=w433) -> ("error out"=w423:errorcluster, "aquisition time ms"=w424:u32, "buffer number"=w390:u32, "captured image"=w418:T4)  [unwired: 5 in]
          n135 = Equal To 0?(x=w377) -> (x = 0?=w432:bool)
          n136 = local read "keyFrameInterval"() -> (w404:i32)
          n137 = Subtract(x=w371, y=w394) -> (x-y=w374:u32)
          "last loop time" <- w374
          n138 = Select(t=w424, s=w432, f=w431) -> (s? t:f=w391:u32)
          n139 = local read "region of interest"() -> (w378:cluster{"x0":u32, "y0":u32, "w":u32, "h":u32})
          n140 = Subtract(x=w424, y=w391) -> (x-y=w416:u32)
          n141 = Quotient & Remainder(x=w377, y=w404) -> (x-y*floor(x/y)=w403:i32, floor(x/y)=w402:i32)
          n142 = call "metadata operations.vi"("add time?"=TRUE, "add to stack writer"=TRUE, "error in (no error)"=w423, "value"=w390, "key"="bufnum", "Operation"=w426) -> ("error out"=w422:errorcluster)  [unwired: 2 in, 3 out]
          n143 = Divide(x=w416, y=u32 1000) -> (x/y=w376:dbl)
          "elapsed time(s)" <- w376
          n144 = Equal To 0?(x=w403) -> (x = 0?=w400:bool)
          n145 = Greater?(x=w402, y=1) -> (0:w399:bool)
          n146 = local read "use ROI"() -> (w379:bool)
          n147 = call "metadata operations.vi"("add time?"=FALSE, "add to stack writer"=TRUE, "error in (no error)"=w422, "value"=w424, "key"="camtime", "Operation"=w426) -> ("error out"=w419:errorcluster)  [unwired: 2 in, 3 out]
          n148 = Greater Or Equal?(x=w376, y="Acquisiton Time (s)") -> (x >= y?=w410:bool)
          n149 = local read "maximum loop time"() -> (w392:u32)
          n150 = Quotient & Remainder(x=w408, y="update image every __ ms") -> (floor(x/y)=w396:u32)  [unwired: 1 out]
          n151 = Not Equal?(x=w396, y=w415) -> (x != y?=w397:bool)
          n152 = And(x=w400, y=w399) -> (x .and. y?=w398:bool)
          n153 = Max & Min(x=w374, y=w392) -> (max(x,y)=→"maximum loop time":u32)  [unwired: 1 out]
          n154 = case shown="False" w379 {
            tunnel: w419 -> [w496 w510]
            tunnel: w418 -> [w495 w514]
            tunnel: w417 -> [w494 w515]
            tunnel: w378 -> [_ w509]
            tunnel: [w493 w513] -> w414
            tunnel: [w492 w511] -> w413
            tunnel: [w491 w512] -> w395
            tunnel: [w490 w497] -> w369
            frame False {
              n155 = call "add IMAQ Frame.vi"("error in (no error)"=w496, "Frame (8 bit 1 channel)"=w495, "Stack Writer In"=w494) -> ("error out"=w493:errorcluster, "frame add time"=w490:u32, "Frame Out"=w491:T4, "Stack Writer Out"=w492:u32)  [unwired: 5 in]
            }
            frame True {
              w498 = T10."Add Value" ("Operation")
              n156 = Unbundle By Name(w509) -> ("x0"=w503:u32, "y0"=w504:u32)
              n157 = call "metadata operations.vi"("add time?"=FALSE, "add to stack writer"=TRUE, "error in (no error)"=w510, "value"=w503, "key"="ROIX", "Operation"=w498) -> ("error out"=w506:errorcluster)  [unwired: 2 in, 3 out]
              n158 = call "metadata operations.vi"("add time?"=FALSE, "add to stack writer"=TRUE, "error in (no error)"=w506, "value"=w504, "key"="ROIY", "Operation"=w498) -> ("error out"=w505:errorcluster)  [unwired: 2 in, 3 out]
              n159 = call "add IMAQ Sub Frame.vi"("error in (no error)"=w505, "subim rectangle"=w509, "Frame (8 bit 1 channel)"=w514, "Stack Writer In"=w515) -> ("error out"=w513:errorcluster, "frame add time"=w497:u32, "Frame Out"=w512:T4, "Stack Writer Out"=w511:u32)  [unwired: 4 in]
            }
          }
          "stackwriter pointer" <- w413
          "frame add time" <- w369
          n160 = case shown="True" w397 {
            tunnel: w395 -> [_ w452]
            tunnel: w379 -> [_ w454]
            tunnel: w378 -> [_ w453]
            frame False {
            }
            frame True {
              n161 = case shown="False" w454 {
                tunnel: w453 -> [_ w460]
                tunnel: w452 -> [w455 w458]
                tunnel: [w455 w456] -> w451
                frame False {
                }
                frame True {
                  n162 = call "IMAQ Clear Overlay"("Image"=w458) -> ("error out"=w459:errorcluster, "Image Out"=w457:T4)  [unwired: 9 in]
                  n163 = call "IMAQ Overlay Rectangle"("error in (no error)"=w459, "Rectangle"=w460, "Image"=w457) -> ("Image Out"=w456:T4)  [unwired: 7 in, 1 out]
                }
              }
              n164 = local write "Camera Image"(w451) -> ()
            }
          }
          n165 = flat-sequence {
            tunnel: w373 -> [w439]
            tunnel: [w439] -> w372
            tunnel: w371 -> [w438]
            tunnel: [w436] -> w370
            frame #0 {
              n166 = local read "keyFrameInterval"() -> (w435:i32)
              n167 = Tick Count (ms)() -> (millisecond timer value=w440:u32)
              n168 = Subtract(x=w440, y=w438) -> (x-y=w437:u32)
              n169 = call <vilib>:"Mean PtByPt.vi"("x"=w437, "sample length"=w435) -> ("mean"=w436:dbl)  [unwired: 2 in, 1 out]
              "average loop time" <- w436
            }
          }
          n170 = local write "buffer number"(w390) -> ()
          n171 = Divide(x=w377, y=w376) -> (x/y=→"avg frame rate (fps)":dbl)
          n172 = case shown="True" w398 {
            tunnel: w414 -> [w461 w488]
            tunnel: w413 -> [_ w473]
            tunnel: [FALSE w477] -> w407
            tunnel: [w461 w463] -> w373
            frame False {
            }
            frame True {
              n173 = call "get Timing Statistics.vi"("error in (no error)"=w488, "sw"=w473) -> ("error out"=w487:errorcluster, "avgWriteTime"=→"average time to write a stack":dbl, "avgCompressTime"=w471:dbl, "avgAddTime"=→"average time to add a frame to stack":dbl)  [unwired: 5 in, 1 out]
              "average time to compress a frame" <- w471
              n174 = Scale By Power Of 2(n=30, x="max stack size") -> (x*2^n=w479:dbl)
              n175 = call "num Bytes Written.vi"("error in (no error)"=w487, "sw"=w473) -> ("error out"=w474:errorcluster, "function return"=w478:i32)  [unwired: 8 in]
              n176 = Greater?(x=w478, y=w479) -> (0:w477:bool)
              n177 = To Double Precision Float(number=w478) -> (double precision float=w480:dbl)
              n178 = Scale By Power Of 2(n=-20, x=w478) -> (x*2^n=→"MB written":i32)
              n179 = Scale By Power Of 2(n=-30, x=w480) -> (x*2^n=→"GB written":dbl)
              n180 = call "get Num Stacks Queued.vi"("error in (no error)"=w474, "sw"=w473) -> ("error out"=w463:errorcluster, "numToWrite"=→"numToWrite":i32, "numToCompress"=w467:i32)  [unwired: 6 in, 1 out]
              "numToCompress" <- w467
              n181 = Multiply(x=100, y=w467) -> (x*y=w465:i32)
              n182 = Add(x=1050.0 ("y"), y=w465) -> (x+y=w464:dbl)
              n183 = Multiply(x=w471, y=w464) -> (x*y=w469:dbl)
              n184 = case shown="True" "auto-set" {
                tunnel: w469 -> [_ w489]
                frame False {
                }
                frame True {
                  n185 = local write "min loop time (ms)"(w489) -> ()
                }
              }
            }
          }
          n186 = Subtract(x="min loop time (ms)", y=w370) -> (x-y=w385:dbl)
          n187 = Greater Than 0?(x=w385) -> (x > 0?=w386:bool)
          "loop too fast" <- w386
          n188 = case shown="False" w386 {
            tunnel: w385 -> [_ w447]
            tunnel: [w443 w445] -> w382
            tunnel: [w444 w446] -> w380
            tunnel: w372 -> [w443 w445]
            frame False {
              n189 = Tick Count (ms)() -> (millisecond timer value=w444:u32)
            }
            frame True {
              n190 = flat-sequence {
                tunnel: [w448] -> _
                tunnel: w447 -> [w450]
                tunnel: [w449] -> w446
                frame #0 {
                  n191 = Tick Count (ms)() -> (millisecond timer value=w448:u32)
                }
                frame #1 {
                  n192 = Wait (ms)(milliseconds to wait=w450) -> (millisecond timer value=w449:u32)
                }
              }
              "delay time" <- w447
            }
          }
          n193 = Unbundle By Name(w382) -> ("status"=w406:bool)
          n194 = Or(x="STOP PROGRAM", y=w406) -> (x .or. y?=w405:bool)
          n195 = Subtract(x=w380, y=w371) -> (x-y=→"total loop\nwith delay":u32)
          n196 = Compound Arithmetic op=OR(w406, "STOP ACQUISITION", w410, w407, "STOP PROGRAM") -> (w409:bool)
        }
        n197 = call "set Num Compression Threads.vi"("error in (no error)"=w296, "maxCompressionThreads"="max Background Compression Threads", "sw"=w240) -> ("error out"=w241:errorcluster)  [unwired: 7 in, 1 out]
        n198 = call "metadata operations.vi"("error in (no error)"=w241, "Operation"=T10."Reset Table") -> ("error out"=w297:errorcluster)  [unwired: 6 in, 3 out]
        n199 = call "metadata operations.vi"("sw"=w240, "error in (no error)"=w297, "Operation"=T10."set stack writer") -> ("error out"=w295:errorcluster)  [unwired: 5 in, 3 out]
        n200 = flat-sequence {
          tunnel: w286 -> [w367]
          tunnel: [w367] -> w285
          frame #0 {
            n201 = local write "maximum loop time"(u32 0 ("maximum loop time")) -> ()
          }
        }
        n202 = property on="region of interest" class="Clust (strict)"(error in=w295, "Visible"=w293) -> (error out=w294:errorcluster)  [unwired: 1 in, 1 out]
        n203 = property on="use ROI" class="Bool (strict)"(error in=w294, "Visible"=w293) -> (error out=w286:errorcluster)  [unwired: 1 in, 1 out]
        n204 = local read "Genotype"() -> (w232:T3)
        n205 = Unbundle By Name(w232) -> ("GAL4 Line / Line A / Genotype"=w231:string, "UAS-Effector Line / Line B"=w230:string)
        n206 = Concatenate Strings(w236, ".dat" ("string")) -> (w276:string)
        n207 = Concatenate Strings(w236, ".speed" ("string")) -> (w269:string)
        n208 = Concatenate Strings(w236, ".git" ("string")) -> (w265:string)
        n209 = Concatenate Strings(w236, ".dlg" ("string")) -> (w262:string)
        n210 = Concatenate Strings(w236, ".notes" ("string")) -> (w257:string)
        n211 = Concatenate Strings(w236, " front panel.jpg" ("string")) -> (w234:string)
        n212 = String To Path(string=w276) -> (path=w275:path)
        n213 = String To Path(string=w269) -> (path=w268:path)
        n214 = String To Path(string=w265) -> (path=w264:path)
        n215 = String To Path(string=w262) -> (path=w261:path)
        n216 = String To Path(string=w257) -> (path=w256:path)
        n217 = String To Path(string=w234) -> (path=w233:path)
        n218 = flat-sequence {
          tunnel: w277 -> [_]
          tunnel: w275 -> [w361]
          tunnel: w268 -> [w358]
          tunnel: w267 -> [w357]
          tunnel: w264 -> [w340]
          tunnel: w261 -> [w355]
          tunnel: [w344] -> w259
          tunnel: w256 -> [w336]
          tunnel: "notes updated: %b %d, %Y, %H:%M" ("time format string (%c)") -> [w335]
          tunnel: w233 -> [w331]
          tunnel: w231 -> [w326]
          tunnel: w230 -> [w325]
          tunnel: w229 -> [w321]
          frame #0 {
            n219 = local read "notes last updated"() -> (w334:timestamp)
            n220 = local read "stimulii"() -> (w327:string[])
            n221 = Build Array (concatenate)("Experimenter" ("notes"), "Experimenter Name", w326, w325, w327) -> (w324:string[])
            n222 = call "get git version.vi"() -> ("error out"=w342:errorcluster, "path to current head"=w341:path)  [unwired: 9 in, 1 out]
            n223 = for {
              tunnel: w324 -> [w366] mode=indexing
              tunnel: [w364] -> w323 mode=indexing
              n224 = Concatenate Strings(w366, "\r\n") -> (w364:string)
            }
            n225 = Copy(8:w342, 10:w340, 11:w341) -> (0:w339:errorcluster)  [unwired: 2 in, 2 out]
            n226 = call "metadata operations.vi"("Operation"=T10."Get Spreadsheet") -> ("error out"=w360:errorcluster, "spreadsheet table"=w362:string)  [unwired: 7 in, 2 out]
            n227 = Format Date/Time String(time format string (%c)=w335, seconds (now)=w334) -> (date/time string=w338:string)  [unwired: 1 in]
            n228 = call <vilib>:"Clear Errors.vi"("error in (no error)"=w339) -> ("error out"=w343:errorcluster)  [unwired: 5 in, 1 out]
            n229 = Write to Text File(file (use dialog)=w361, text=w362, error in=w360) -> (error out=w359:errorcluster)  [unwired: 1 in, 2 out]
            n230 = Write to Text File(file (use dialog)=w358, text=w357, error in=w359) -> (error out=w346:errorcluster)  [unwired: 1 in, 2 out]
            n231 = Concatenate Strings(w323, w338, "\r\n", "notes") -> (w318:string)
            n232 = control-ref of="This VI"() -> (w332:refnum<vi>)
            n233 = Equal?(x="notes", y=w321) -> (x = y?=w320:bool)
            n234 = invoke class="VI" method="Ctrl Val.Get All"(reference=w332, "Controls"=TRUE) -> (error out=w354:errorcluster, "Get All Control Values Variant"=w349:cluster{"Name":string, "Variant Data":variant}[])  [unwired: 2 in, 2 out]
            n235 = Open/Create/Replace Datalog(5:w349, 8:w354, 9:enum16{"read/write", "read-only", "write-only"}."write-only" ("access (0:read/write)"), 10:T11."replace or create" ("operation (0:open)"), 11:w355) -> (0:w351:errorcluster, 3:w350:refnum<k1>)  [unwired: 1 in, 1 out]
            n236 = Concatenate Strings(w318, "\r\n", "notes updated during recording" ("string")) -> (w319:string)
            n237 = Select(t=w318, s=w320, f=w319) -> (s? t:f=w317:string)
            n238 = Write Datalog(4:w351, 6:w349, 7:w350) -> (0:w348:errorcluster, 3:w347:refnum<k1>)
            n239 = Write to Text File(file (use dialog)=w336, text=w317) -> (error out=w333:errorcluster)  [unwired: 2 in, 2 out]
            n240 = call "save vi front panel image.vi"("path to JPEG file"=w331, "This VI"=w332) -> ("error out"=w330:errorcluster)  [unwired: 9 in]
            n241 = Close File(refnum=w347, error in=w348) -> (error out=w345:errorcluster)  [unwired: 1 out]
            n242 = Build Array(w346, w343, w345, w333, w330) -> (w344:errorcluster[])
          }
        }
        n243 = call "metadata operations.vi"("sw"=u32 0, "error in (no error)"=w251, "Operation"=T10."set stack writer") -> ("error out"=w250:errorcluster)  [unwired: 5 in, 3 out]
        n244 = call <vilib>:"Clear Errors.vi"("error in (no error)"=w250) -> ("error out"=w247:errorcluster)  [unwired: 5 in, 1 out]
        n245 = call "stop Recording.vi"("error in (no error)"=w247, "sw"=w254) -> ("error out"=w274:errorcluster, "sw out"=w272:u32)  [unwired: 7 in, 1 out]
        n246 = call "flag experiment state.vi"("error in (no error)"=w247, "experiment started"=FALSE) -> ("error out"=w245:errorcluster)  [unwired: 9 in]
        n247 = call "get Timing Report.vi"("error in (no error)"=w274, "maxchars"=65536, "sw"=w272) -> ("error out"=w273:errorcluster, "dst"=w267:string)  [unwired: 6 in, 1 out]
        "timing report" <- w267
        n248 = call "destroy Stack Writer.vi"("error in (no error)"=w273, "sw"=w272) -> ("error out"=w288:errorcluster)  [unwired: 9 in]
        n249 = Merge Errors(w251, w288, w245) -> (w284:errorcluster)
        n250 = property on="use ROI" class="Bool (strict)"(error in=w284, "Visible"=w283) -> (error out=w280:errorcluster)  [unwired: 1 in, 1 out]
        n251 = property on="region of interest" class="Clust (strict)"(error in=w280, "Visible"=w283) -> (error out=w281:errorcluster)  [unwired: 1 in, 1 out]
        n252 = property on="STOP ACQUISITION" class="Bool"(error in=w281, "Visible"=FALSE) -> (error out=w279:errorcluster)  [unwired: 1 in, 1 out]
        n253 = Merge Errors(w279, w259) -> (w260:errorcluster)
      }
      event "set all control values as default": Mouse Up {
        # "experiment description default values bin file"
        # "vi name"
        n254 = event-data() -> ()  [unwired: 1 in, 8 out]
        n255 = control-ref of="This VI"() -> (w539:refnum<vi>)
        n256 = invoke class="VI" method="Ctrl Val.Get All"(reference=w539, error in=w538, "Controls"=TRUE) -> (error out=w530:errorcluster, "Get All Control Values Variant"=w523:cluster{"Name":string, "Variant Data":variant}[])  [unwired: 1 in, 2 out]
        n257 = Current VI's Path() -> (path=w517:path)
        n258 = call <vilib>:"Get File Extension.vi"("file"=w517) -> ("filename without extension"=w516:string)  [unwired: 6 in, 4 out]
        n259 = Strip Path(path=w517) -> (stripped path=w536:path)  [unwired: 1 out]
        n260 = Strip Path(path=w536) -> (stripped path=w535:path)  [unwired: 1 out]
        n261 = Concatenate Strings(w516, " ctl values.dflt" ("string")) -> (w531:string)
        n262 = File/Directory Info(path=w536, error in=w530) -> (directory=w534:bool, error out=w529:errorcluster)  [unwired: 5 out]
        n263 = Select(t=w536, s=w534, f=w535) -> (s? t:f=w532:path)
        n264 = Build Path(base path=w532, name or relative path=w531) -> (appended path=w528:path)
        n265 = Open/Create/Replace Datalog(5:w523, 8:w529, 9:enum16{"read/write", "read-only", "write-only"}."write-only" ("access (0:read/write)"), 10:T11."replace or create" ("operation (0:open)"), 11:w528) -> (0:w525:errorcluster, 3:w524:refnum<k1>)  [unwired: 1 in, 1 out]
        n266 = Write Datalog(4:w525, 6:w523, 7:w524) -> (0:w522:errorcluster, 3:w521:refnum<k1>)
        n267 = Close File(refnum=w521, error in=w522) -> (error out=w519:errorcluster)  [unwired: 1 out]
        n268 = Unbundle By Name(w519) -> ("status"=w518:bool)
      }
      event "save control values to file": Mouse Up {
        # "experiment description default values bin file"
        n269 = event-data() -> ()  [unwired: 1 in, 8 out]
        n270 = control-ref of="This VI"() -> (w565:refnum<vi>)
        n271 = invoke class="VI" method="Ctrl Val.Get All"(reference=w565, error in=w564, "Controls"=TRUE) -> (error out=w558:errorcluster, "Get All Control Values Variant"=w556:cluster{"Name":string, "Variant Data":variant}[])  [unwired: 1 in, 2 out]
        n272 = local read "Experimenter Name"() -> (w544:string)
        n273 = Current VI's Path() -> (path=w552:path)
        n274 = Format Date/Time String(time format string (%c)="%Y%m%d") -> (date/time string=w543:string)  [unwired: 2 in]
        n275 = Strip Path(path=w552) -> (stripped path=w562:path)  [unwired: 1 out]
        n276 = Concatenate Strings(w544, w543, ".dlg" ("element")) -> (w541:string)
        n277 = Strip Path(path=w562) -> (stripped path=w561:path)  [unwired: 1 out]
        n278 = File/Directory Info(path=w562, error in=w558) -> (directory=w560:bool, error out=w547:errorcluster)  [unwired: 5 out]
        n279 = Select(t=w562, s=w560, f=w561) -> (s? t:f=w559:path)
        n280 = Build Path(base path=w559, name or relative path="user settings") -> (appended path=w557:path)
        n281 = call "File Dialog"("start path"=w557, "prompt"="select or create dlg file to save control values", "default name"=w541, "error in"=w547, "pattern (all files)"="*.dlg") -> ("selected path"=w550:path, "cancelled"=w540:bool, "error out"=w546:errorcluster)  [unwired: 7 in, 1 out]
        n282 = case shown="True" w540 {
          tunnel: w556 -> [w571 _]
          tunnel: [w568 w576] -> w554
          tunnel: w550 -> [w567 _]
          tunnel: w546 -> [w566 w576]
          frame False {
            n283 = Open/Create/Replace Datalog(5:w571, 8:w566, 9:enum16{"read/write", "read-only", "write-only"}."write-only" ("access (0:read/write)"), 10:T11."replace or create" ("operation (0:open)"), 11:w567) -> (0:w573:errorcluster, 3:w572:refnum<k1>)  [unwired: 1 in, 1 out]
            n284 = Write Datalog(4:w573, 6:w571, 7:w572) -> (0:w570:errorcluster, 3:w569:refnum<k1>)
            n285 = Close File(refnum=w569, error in=w570) -> (error out=w568:errorcluster)  [unwired: 1 out]
          }
          frame True {
          }
        }
        n286 = Unbundle By Name(w554) -> ("status"=w553:bool)
      }
      event "load control values from file": Mouse Up {
        # "cause event 1 to fire"
        # "experiment description default values bin file"
        n287 = event-data() -> ()  [unwired: 1 in, 8 out]
        n288 = Current VI's Path() -> (path=w593:path)
        n289 = Strip Path(path=w593) -> (stripped path=w600:path)  [unwired: 1 out]
        n290 = Strip Path(path=w600) -> (stripped path=w599:path)  [unwired: 1 out]
        n291 = File/Directory Info(path=w600, error in=w585) -> (directory=w598:bool, error out=w588:errorcluster)  [unwired: 5 out]
        n292 = Select(t=w600, s=w598, f=w599) -> (s? t:f=w597:path)
        n293 = Build Path(base path=w597, name or relative path="user settings") -> (appended path=w596:path)
        n294 = call "File Dialog2"("start path"=w596, "prompt"="select dlg file to load control values", "error in"=w588, "pattern (all files)"="*.dlg") -> ("selected path"=w591:path, "cancelled"=w586:bool, "error out"=w587:errorcluster)  [unwired: 8 in, 1 out]
        n295 = control-ref of="Edit"() -> (w582:refnum<vi>)
        n296 = control-ref of="Delete"() -> (w583:refnum<vi>)
        n297 = control-ref of="stimulii"() -> (w584:refnum<vi>)
        n298 = case shown="False" w586 {
          tunnel: [w604 w617] -> w577
          tunnel: w591 -> [w607 _]
          tunnel: w587 -> [w608 w617]
          tunnel: w584 -> [w603 _]
          tunnel: w583 -> [w602 _]
          tunnel: w582 -> [w601 _]
          frame False {
            n299 = control-ref of="This VI"() -> (w606:refnum<vi>)
            n300 = call "load control values from file.vi"("error in (no error)"=w608, "datalog path (use dialog)"=w607, "VI ref"=w606) -> ("error out"=w605:errorcluster)  [unwired: 8 in]
            n301 = flat-sequence {
              tunnel: w605 -> [w616]
              tunnel: [w614] -> w604
              tunnel: w603 -> [w612]
              tunnel: w602 -> [w611]
              tunnel: w601 -> [w610]
              frame #0 {
                n302 = local read "Stimulus Array"() -> (w609:T2)
                n303 = call "stimulus params to string gershow.vi"("Stimulus cluster array"=w609, "error in"=w616) -> ("error out"=w615:errorcluster, "long string array"=w613:string[])  [unwired: 5 in, 3 out]
                n304 = local write "stimulii"(w613) -> ()
                n305 = call "adjust stimulus buttons.vi"("Stimulus Array"=w609, "error in (no error)"=w615, "Edit handle"=w610, "Delete handle"=w611, "stimulii handle"=w612) -> ("error out"=w614:errorcluster)  [unwired: 6 in]
              }
            }
          }
          frame True {
          }
        }
        n306 = property class="Arr"(reference=w582, error in=w577) -> (reference out=w581:refnum<vi>, error out=w579:errorcluster, "Value"=w580:variant)
        n307 = property class="Arr"(reference=w581, error in=w579, "Val(Sgnl)"=w580) -> (error out=w578:errorcluster)  [unwired: 1 out]
        n308 = Unbundle By Name(w578) -> ("status"=w594:bool)
      }
      event "STOP PROGRAM": Mouse Up {
        n309 = event-data() -> ()  [unwired: 1 in, 8 out]
      }
      event "MAKE DIRECTORIES": Mouse Up {
        n310 = event-data() -> ()  [unwired: 1 in, 8 out]
        n311 = local read "Genotype"() -> (w624:T3)
        n312 = local read "Training/Habituation Pre Exposure"() -> (w627:T1)
        n313 = local read "Stimulus Array"() -> (w625:T2)
        n314 = local read "Project"() -> (w626:string)
        n315 = local read "use short dir"() -> (w621:bool)
        n316 = call "experiment description to file name Gershow.vi"("use short dir"=w621, "Training/Habituation Pre Exposure"=w627, "error in"=w623, "Stimulus Array"=w625, "Genotype"=w624, "Project"=w626) -> ("error out"=w622:errorcluster, "data directory with time"=w636:path, "filename"=w635:string)  [unwired: 2 in, 1 out]
        n317 = local write "filename"(w635) -> ()
        n318 = Build Path(base path="base directory", name or relative path=w636) -> (appended path=w628:path)
        n319 = local write "data directory"(w628) -> ()
        n320 = call <vilib>:"Check if File or Folder Exists.vi"("error in (no error)"=w622, "path"=w628) -> ("error out"=w638:errorcluster, "file or folder exists?"=w637:bool, "dup path"=w639:path)  [unwired: 7 in]
        n321 = case shown="False" w637 {
          tunnel: w639 -> [w645 w651]
          tunnel: w638 -> [w644 w652]
          tunnel: [w643 w650] -> w633
          tunnel: "directory already exists and is not empty" ("message") -> [_ w648]
          tunnel: [TRUE w646] -> w632
          frame False {
            n322 = Create Folder(path (use dialog)=w645, error in=w644) -> (error out=w643:errorcluster)  [unwired: 1 in, 2 out]
          }
          frame True {
            n323 = call <vilib>:"Recursive File List.vi"("error in (no error)"=w652, "Folder Path"=w651) -> ("error out"=w650:errorcluster, "Number of Files"=w649:i32)  [unwired: 5 in, 3 out]
            n324 = Greater Than 0?(x=w649) -> (x > 0?=w647:bool)
            n325 = case shown="True" w647 {
              tunnel: w648 -> [_ w653]
              frame False {
              }
              frame True {
                n326 = One Button Dialog(message=w653) -> ()  [unwired: 1 in, 1 out]
              }
            }
            n327 = Not(x=w647) -> (.not. x?=w646:bool)
          }
        }
        n328 = control-ref of="START ACQUISITION"() -> (w641:refnum<vi>)
        n329 = property class="Bool (strict)"(reference=w641, error in=w633, "Visible"=w632) -> (error out=w629:errorcluster)  [unwired: 1 out]
        n330 = Unbundle By Name(w629) -> ("status"=w630:bool)
      }
      event "notes": Value Change {
        n331 = event-data() -> ()  [unwired: 1 in, 6 out]
        n332 = Get Date/Time In Seconds() -> (seconds since 1Jan1904=→"notes last updated":timestamp)
      }
    }
    "loop iteration" <- w72
  }
  "error out" <- w28
  n333 = call <vilib>:"Clear Errors.vi"("error in (no error)"=w28) -> ("error out"=w30:errorcluster)  [unwired: 5 in, 1 out]
  n334 = call "close image source.vi"("error in (no error)"=w30, "image source data"=w31) -> ("error out"=w29:errorcluster)  [unwired: 9 in]
  n335 = Merge Errors(w28, w29) -> (w27:errorcluster)
  n336 = call <vilib>:"Simple Error Handler.vi"("type of dialog (OK msg:1)"=w26, "error in (no error)"=w27) -> ()  [unwired: 3 in, 5 out]
